vi "Single Read of Counter Value.vi"() -> ()   [LabVIEW 2020]
uses:
  <instrlib>/BDAQ-6104/Private/Edge Triger Type.ctl
  <instrlib>/BDAQ-6104/Public/Configure/Configure Edge Counter.vi
  <instrlib>/BDAQ-6104/Public/Data/Start Counter.vi
  <instrlib>/BDAQ-6104/Public/Data/Read Counter Value.vi
  <instrlib>/BDAQ-6104/Public/Data/Stop Counter.vi
  <instrlib>/BDAQ-6104/BDAQ-6104.lvlib
panel:
  in  "Mode":T1=enum."RISING"
  in  "milliseconds to wait":u32=1000
  out "Count":i32
  in  "VISA resource name":refnum<visa-resource-name>
  # "In this example, a delay is introduced to \nallow a mechanism to generate an edge signal.\nThis could be a button or other signal source."
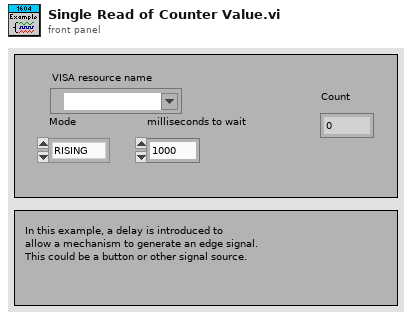
[diagram p1: front panel]
types:
  T1 = typedef "BDAQ-6104.lvlib/Edge Triger Type.ctl" = enum16{"CHANGE", "FALLING", "RISING"}
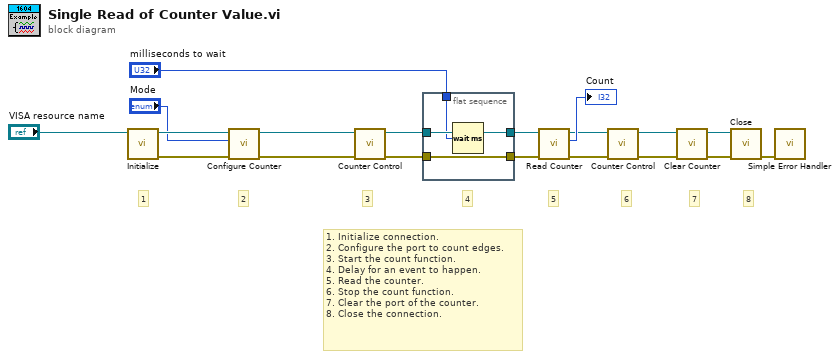
[diagram p0: block diagram]
diagram:
  # "1. Initialize connection.\n2. Configure the port to count edges.\n3. Start the count function.\n4. Delay for an event to happen.\n5. Read the counter.\n6. Stop the count function.\n7. Clear the port of the counter.\n8. Close the connection."
  # "8"
  # "7"
  # "6"
  # "5"
  # "4"
  # "3"
  # "2"
  # "1"
  n1 = call <instrlib>:"Initialize.vi"("VISA resource name"="VISA resource name") -> ("error out"=w17:errorcluster, "VISA resource name out"=w18:refnum<visa-resource-name>)  [unwired: 9 in]
  n2 = call-poly <instrlib>:"Configure Counter.vi"("error in"=w17, "Mode"="Mode", "VISA resource name"=w18) -> ("error out"=w14:errorcluster, "VISA resource name out"=w13:refnum<visa-resource-name>)  [unwired: 7 in]
  n3 = call-poly <instrlib>:"Counter Control.vi"("error in (no error)"=w14, "VISA resource name"=w13) -> ("error out"=w10:errorcluster, "VISA resource name out"=w8:refnum<visa-resource-name>)  [unwired: 8 in]
  n4 = flat-sequence {
    tunnel: w10 -> [w22]
    tunnel: [w22] -> w9
    tunnel: [w21] -> w7
    tunnel: w8 -> [w21]
    tunnel: "milliseconds to wait" -> [w20]
    frame #0 {
      n5 = Wait (ms)(milliseconds to wait=w20) -> ()  [unwired: 1 out]
    }
  }
  n6 = call-poly <instrlib>:"Read Counter.vi"("error in (no error)"=w9, "VISA resource name"=w7) -> ("error out"=w11:errorcluster, "Count"=→"Count":i32, "VISA resource name out"=w12:refnum<visa-resource-name>)  [unwired: 7 in]
  n7 = call-poly <instrlib>:"Counter Control.vi"("error in (no error)"=w11, "VISA resource name"=w12) -> ("error out"=w4:errorcluster, "VISA resource name out"=w2:refnum<visa-resource-name>)  [unwired: 8 in]
  n8 = call <instrlib>:"Clear Counter.vi"("error in (no error)"=w4, "VISA resource name"=w2) -> ("error out"=w3:errorcluster, "VISA resource name out"=w1:refnum<visa-resource-name>)  [unwired: 8 in]
  n9 = call <instrlib>:"Close.vi"("error in (no error)"=w3, "VISA resource name"=w1) -> ("error out"=w16:errorcluster)  [unwired: 9 in]
  n10 = call <vilib>:"Simple Error Handler.vi"("error in (no error)"=w16) -> ()  [unwired: 4 in, 5 out]
